vi "Create Sessions - 1Sess.vi"(7 "option string":string, 8 "error in":errorcluster, 9 "reset":bool, 11 "session reservation in":refnum<class "Session Reservation.lvclass">) -> (0 "error out":errorcluster, 1 "channel list":string, 2 "session":refnum<k15>, 3 "session reservation out":refnum<class "Session Reservation.lvclass">)   [LabVIEW 2020, in "MeasurementLink niDMM.lvlib"]
doc: "Create the NI-DMM driver session from a reservation. Returns an error if more than one NI-DMM session has been reserved. Use \"Create Session - NSess.vi\" for multiple sessions."
uses:
  MeasurementLink Session Management/Session Reservation/Session Reservation.lvclass
  7f77feb2-d2b5-4acd-8f0f-f1b24b7d1641.vi
  Instrument/Instrument.lvclass
  C:/Users/lvadmin/Desktop/measurementlink-labview/Source/Runtime/MeasurementLink Instrument/IInstrument/IInstrument.lvclass
  MeasurementLink Session Management/Session Reservation/Create Sessions Impl.vi
  MeasurementLink niDMM.lvlib
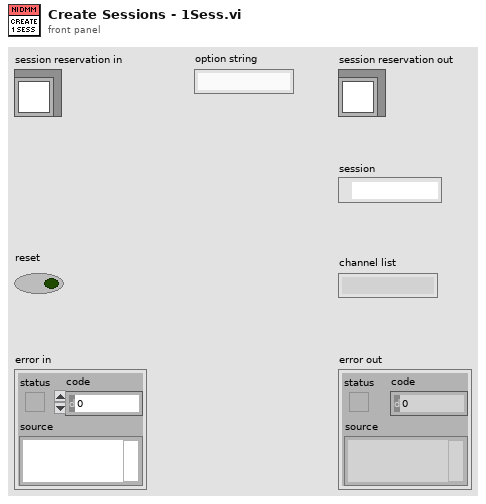
[diagram p1: front panel]
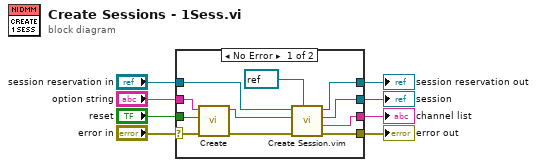
[diagram p0: block diagram]
diagram:
  n1 = case shown="No Error" "error in" {
    selector: "error in" -> [w12 w21]
    tunnel: [w18 w21] -> w7
    tunnel: [w19 w20] -> w5
    tunnel: "session reservation in" -> [w14 w20]
    tunnel: "option string" -> [w10 _]
    tunnel: "reset" -> [w11 _]
    tunnel: [w17 _] -> w2
    tunnel: [w16 _] -> w1
    frame No Error {
      n2 = call "Create.vi"("error in"=w12, "reset"=w11, "option string"=w10) -> ("error out"=w13:errorcluster, "instrument out"=w9:refnum<class "Instrument.lvclass">)  [unwired: 7 in]
      n3 = call "Create Session.vim"("session type"=refnum<k15> refnum ("instrument handle out"), "error in"=w13, "instrument"=w9, "session reservation in"=w14) -> ("error out"=w18:errorcluster, "channel list"=w17:string, "session"=w16:refnum<k15>, "session reservation out"=w19:refnum<class "Session Reservation.lvclass">)  [unwired: 4 in]
    }
    frame Error {
    }
  }
  "error out" <- w7
  "session reservation out" <- w5
  "session" <- w1
  "channel list" <- w2
